vi "ReadJSONSingleNumberFromDevice.vi"(8 "error":errorcluster, 9 "timed out?":bool, 10 "JSON Key of Interest":string="$.results", 11 "JSON reply":string) -> (0 "error out":errorcluster, 1 "Found":bool, 3 "Data":i32)   [LabVIEW 2023, in "GenericDevice.lvclass"]
uses:
  GenericDevice.lvclass
  183c3eef-430e-49c4-ac70-65617c8266b1.vi
  <vilib>/JDP Science/JSONtext/Find Item.vi
  <vilib>/JDP Science/JSONtext/Next JSON Value.vi
  <vilib>/JDP Science/JSONtext/String Subset.vi
  <vilib>/JDP Science/JSONtext/Parsing/Advance past next JSON Value (inlined COPY).vi
  <vilib>/JDP Science/JSONtext/Parsing/Advance past whitespace.vi
  <vilib>/JDP Science/JSONtext/Parsing/Advance past String.vi
  <vilib>/JDP Science/JSONtext/Parsing/Advance past Number.vi
  <vilib>/JDP Science/JSONtext/Parsing/Advance past Line Ending.vi
  <vilib>/JDP Science/JSONtext/Parsing/Parse Full Path or Item Name.vi
  <vilib>/JDP Science/JSONtext/Parsing/Advance past Array.vi
  <vilib>/JDP Science/JSONtext/Parsing/Advance past Object.vi
  <vilib>/JDP Science/JSONtext/support/Error Cluster From Code.vi
  <vilib>/JDP Science/JSONtext/Offset/Find Item Locations by Path.vi
  <vilib>/JDP Science/JSONtext/JSON text to Variant.vi
  <vilib>/JDP Science/JSONtext/LVClass Serializer/JSONtext LVClass Serializer.lvclass
  GenericDevice.lvclass/GenericDevice.ctl
panel:
  # "Connector Pane"
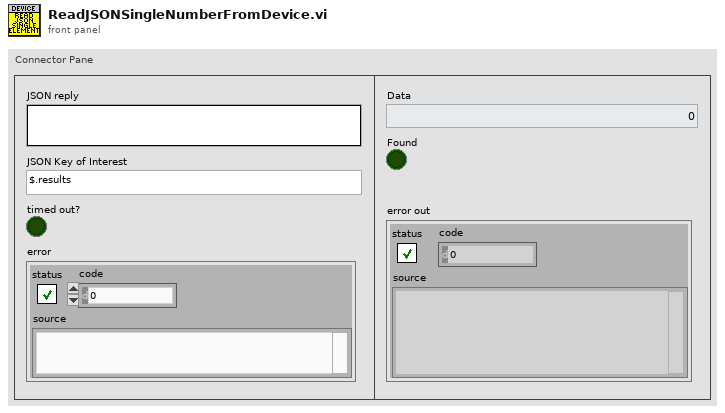
[diagram p1: front panel]
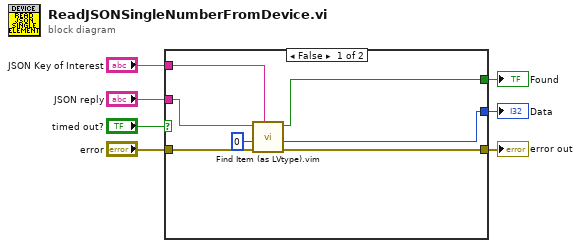
[diagram p0: block diagram]
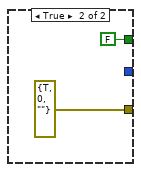
[diagram p2: hidden frame]
diagram:
  n1 = case shown="False" "timed out?" {
    tunnel: [w13 errorcluster {"status"=TRUE, "code"=0, "source"=""} ("error")] -> w3
    tunnel: "error" -> [w14 _]
    tunnel: "JSON reply" -> [w10 _]
    tunnel: "JSON Key of Interest" -> [w11 _]
    tunnel: [w12 _] -> w2
    tunnel: [w8 FALSE ("Found")] -> w1
    frame False {
      n2 = call "Find Item (as LVtype).vim"("$Path or Item Name"=w11, "error in (no error)"=w14, "Data Type and Default Value"=0, "JSON"=w10) -> ("error out"=w13:errorcluster, "Data"=w12:i32, "Found"=w8:bool)  [unwired: 4 in, 1 out]
    }
    frame True {
    }
  }
  "error out" <- w3
  "Data" <- w2
  "Found" <- w1
